vi "BallDispPosSkillVSS.vi"(8 "error in (no error)":errorcluster, 9 "Game":refnum<class "Game.lvclass">, 10 "Robot in":refnum<class "Robot.lvclass">, 11 "BallDispPosSkillVSS in":refnum<class "BallDispPosSkillVSS.lvclass">) -> (0 "error out":errorcluster, 2 "Robot out":refnum<class "Robot.lvclass">, 3 "BallDispPosSkillVSS out":refnum<class "BallDispPosSkillVSS.lvclass">)   [LabVIEW 2020, in "BallDispPosSkillVSS.lvclass"]
uses:
  BallDispPosSkillVSS.lvclass
  Robot_class/Robot.lvclass
  Game_class/Game.lvclass
  Ball_class/Ball.lvclass
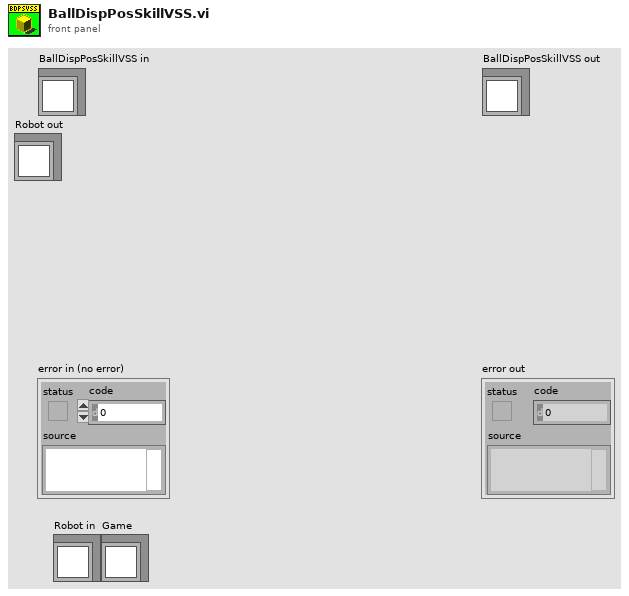
[diagram p1: front panel]
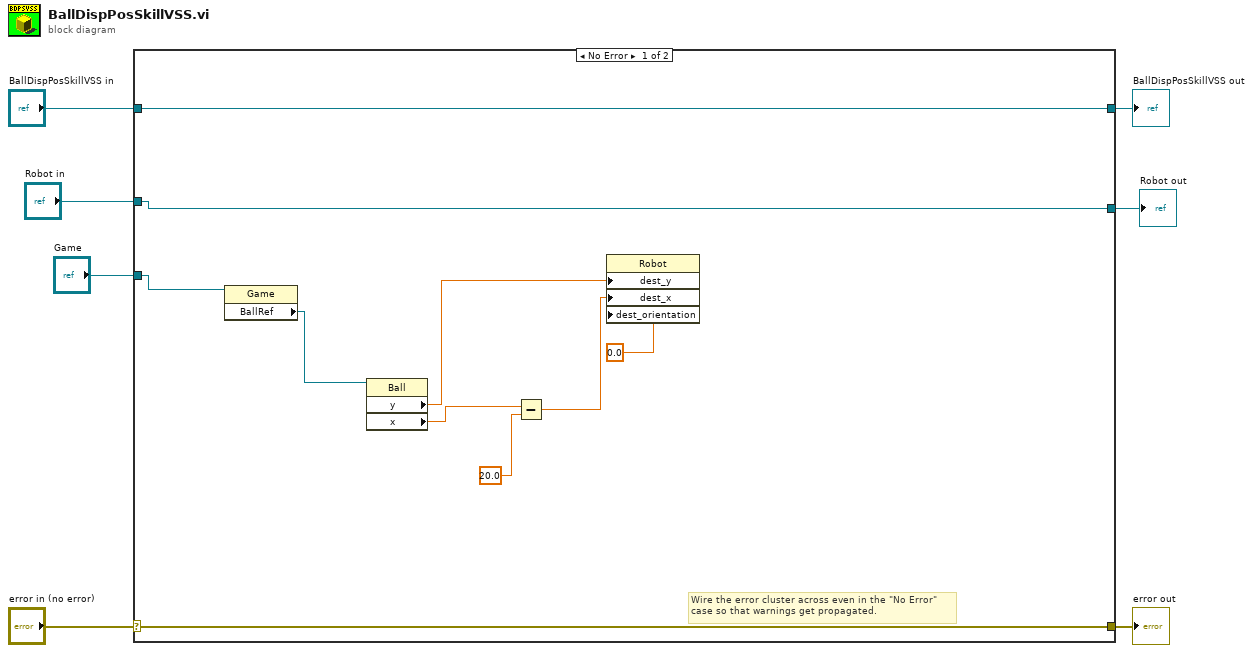
[diagram p0: block diagram]
diagram:
  n1 = case shown="No Error" "error in (no error)" {
    selector: "error in (no error)" -> [w16 w19]
    tunnel: [w16 w19] -> w6
    tunnel: [w17 w18] -> w4
    tunnel: "BallDispPosSkillVSS in" -> [w17 w18]
    tunnel: "Robot in" -> [w15 _]
    tunnel: "Game" -> [w9 _]
    tunnel: [w15 _] -> w1
    frame No Error {
      # "Wire the error cluster across even in the \"No Error\"\ncase so that warnings get propagated."
      n2 = property class="Game"(reference=w9) -> ("BallRef"=w8:refnum<class "Ball.lvclass">)  [unwired: 1 in, 2 out]
      n3 = property class="Ball"(reference=w8) -> ("y"=w10:dbl, "x"=w12:dbl)  [unwired: 1 in, 2 out]
      n4 = Subtract(x=w12, y=20.0) -> (x-y=w11:dbl)
      n5 = property class="Robot"("dest_y"=w10, "dest_x"=w11, "dest_orientation"=0.0) -> ()  [unwired: 2 in, 2 out]
    }
    frame Error {
    }
  }
  "error out" <- w6
  "BallDispPosSkillVSS out" <- w4
  "Robot out" <- w1
